vi "clearpath_close.vi"(0 "ClearpathComm":T1) -> ()   [LabVIEW 2012, in "clearpath_interface.lvlib"]
doc: "Closes Clearpath Robotics interface (destroys queues, closes serial port)"
uses:
  IGVC/Clearpath/Husky 2011/Teleop Robotics Project Folder/Husky/vi/clearpath_interface.lvlib
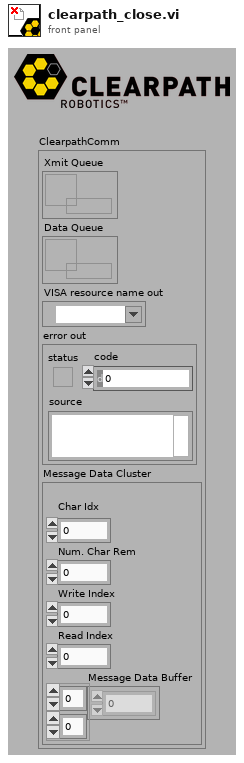
[diagram p1: front panel]
types:
  T1 = cluster{"Xmit Queue":refnum<queue>, "Data Queue":refnum<queue>, "VISA resource name out":refnum<visa-resource-name>, "error out":errorcluster, "Message Data Cluster":cluster{"\nChar Idx":u8, "Num. Char Rem":u8, "Write Index":u8, "Read Index":u8, "Message Data Buffer":u8[][]}}
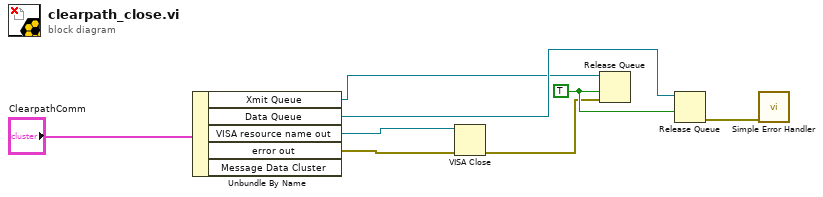
[diagram p0: block diagram]
diagram:
  w6 = TRUE ("force destroy? (F)")
  n1 = Unbundle By Name("ClearpathComm") -> ("Xmit Queue"=w5:refnum<queue>, "Data Queue"=w7:refnum<queue>, "VISA resource name out"=w3:refnum<visa-resource-name>, "error out"=w4:errorcluster)  [unwired: 1 out]
  n2 = VISA Close(VISA resource name=w3, error in (no error)=w4) -> (error out=w2:errorcluster)
  n3 = Release Queue(queue=w5, force destroy? (F)=w6, error in (no error)=w2) -> ()  [unwired: 3 out]
  n4 = Release Queue(queue=w7, force destroy? (F)=w6) -> (error out=w8:errorcluster)  [unwired: 1 in, 2 out]
  n5 = call <vilib>:"Simple Error Handler.vi"("error in (no error)"=w8) -> ()  [unwired: 4 in, 5 out]
